vi "test - Add VI Reference Script.vi"(8 "error in (no error)":errorcluster, 11 "TestCase in":refnum<class "testcase-csmhelper.lvclass">) -> (0 "error out":errorcluster, 3 "TestCase out":refnum<class "testcase-csmhelper.lvclass">)   [LabVIEW 2017, in "testcase-csmhelper.lvclass"]
uses:
  testcase-csmhelper.lvclass
  src/user.lib/_NEVSTOP/Communicable State Machine(CSM)/_csmHelper/CSM-Helper.lvclass/CSM-Helper.ctl
  src/user.lib/_NEVSTOP/Communicable State Machine(CSM)/_csmHelper/Properties/Read VI Ref.vi
  src/user.lib/_NEVSTOP/Communicable State Machine(CSM)/_csmHelper/API/Create From VI Reference.vi
  src/user.lib/_NEVSTOP/Communicable State Machine(CSM)/_csmHelper/API/Open Block Diagram.vi
  src/user.lib/_NEVSTOP/Communicable State Machine(CSM)/_csmHelper/API/Start Undo.vi
  src/user.lib/_NEVSTOP/Communicable State Machine(CSM)/_csmHelper/API/Remove State Frame.vi
  src/user.lib/_NEVSTOP/Communicable State Machine(CSM)/_csmHelper/usecase/Add VI Reference Case.vi
  src/user.lib/_NEVSTOP/Communicable State Machine(CSM)/_csmHelper/API/Stop Undo.vi
  src/user.lib/_NEVSTOP/Communicable State Machine(CSM)/_csmHelper/Properties/Read States.vi
  src/user.lib/_NEVSTOP/Communicable State Machine(CSM)/_csmHelper/API/Undo.vi
  src/user.lib/_NEVSTOP/Communicable State Machine(CSM)/_csmHelper/API/Destroy.vi
  <vilib>/addons/_JKI Toolkits/VI Tester/TestCase.llb/TestCase.lvclass
  src/user.lib/_NEVSTOP/Communicable State Machine(CSM)/_csmHelper/CSM-Helper.lvclass
  C:/Program Files (x86)/National Instruments/LabVIEW 2017/vi.lib/addons/_JKI Toolkits/VI Tester/TestCase.llb/TestCase.lvclass
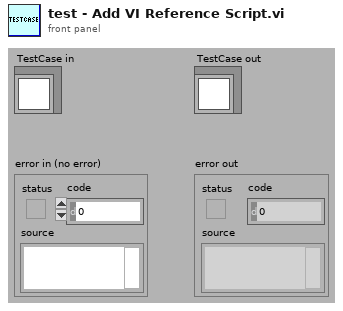
[diagram p1: front panel]
types:
  T1 = enum32{"Bad", "Idle", "Run top level", "Running"}
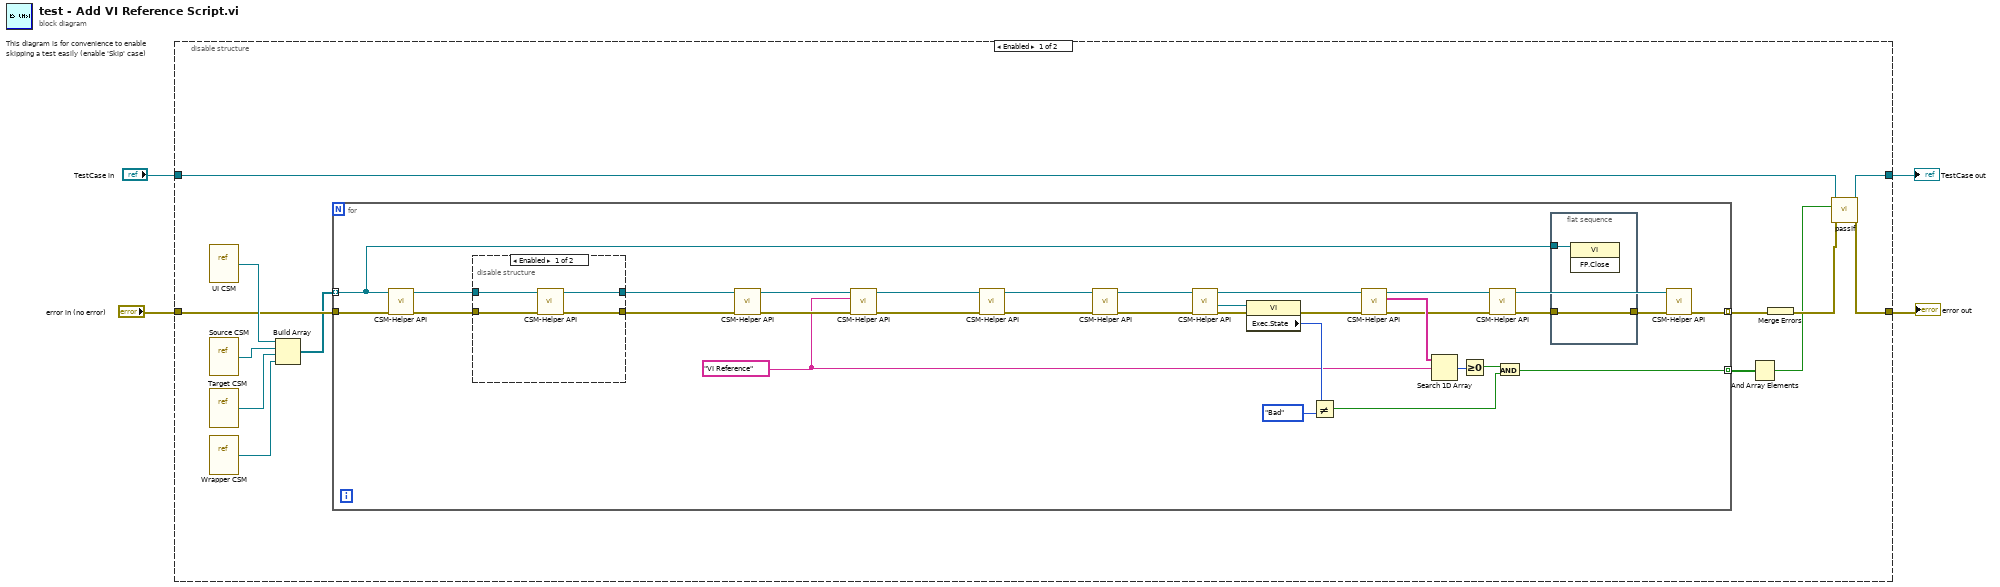
[diagram p0: block diagram]
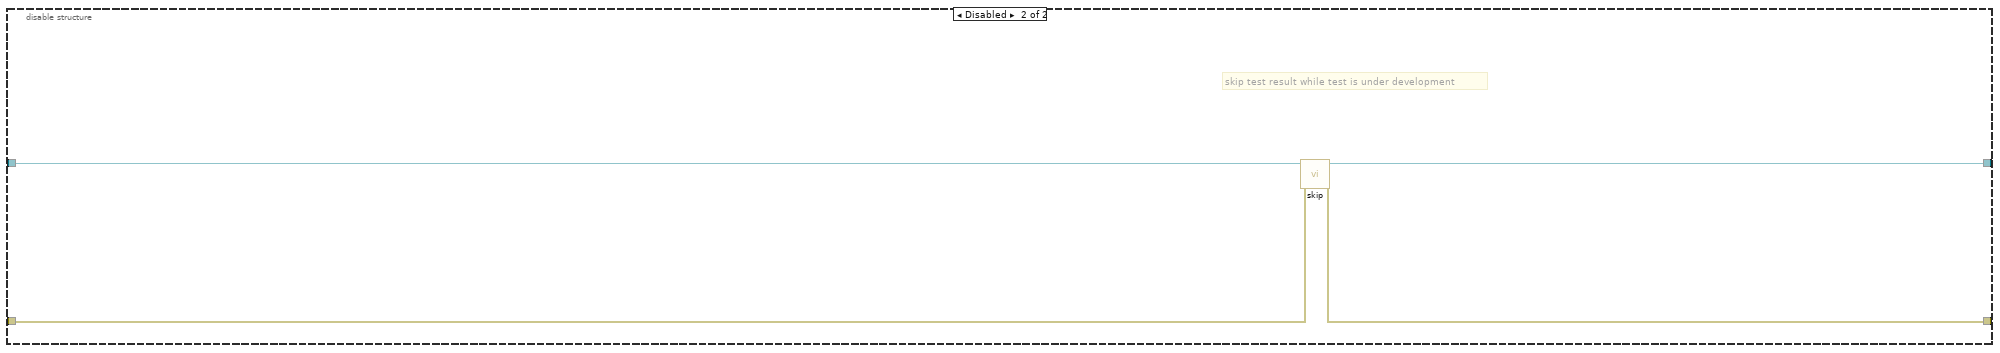
[diagram p3: hidden frame]
diagram:
  n1 = disable-structure "This diagram is for convenience to enable skipping a test easily (enable 'Skip' case)" shown="Enabled" {
    disable-tunnel: "TestCase in" -> [w17 w61]
    disable-tunnel: [w16 w59] -> w1
    disable-tunnel: [w15 w60] -> w3
    disable-tunnel: "error in (no error)" -> [w12 w58]
    frame Enabled {
      n2 = vi-ref "UI CSM.vi"() -> (w14:refnum<vi>)
      n3 = vi-ref "Source CSM.vi"() -> (w8:refnum<vi>)
      n4 = vi-ref "Target CSM.vi"() -> (w7:refnum<vi>)
      n5 = vi-ref "Wrapper CSM.vi"() -> (w6:refnum<vi>)
      n6 = Build Array(w14, w8, w7, w6) -> (w5:refnum<vi>[])
      n7 = for {
        tunnel: w5 -> [w20] mode=indexing
        tunnel: [w49] -> w13 mode=indexing
        tunnel: w12 -> [w48]
        tunnel: [w47] -> w11 mode=indexing
        w21 = "VI Reference" ("element")
        n8 = call-poly "CSM-Helper API.vi"("error in (no error)"=w48, "VI"=w20) -> ("error out"=w25:errorcluster, "CSM-Helper.lvclass"=w24:refnum<class "CSM-Helper.lvclass">)  [unwired: 8 in]
        n9 = disable-structure shown="Enabled" {
          disable-tunnel: w25 -> [w55 w56]
          disable-tunnel: w24 -> [w54 w57]
          disable-tunnel: [w53 w56] -> w23
          disable-tunnel: [w52 w57] -> w22
          frame Enabled {
            n10 = call-poly "CSM-Helper API.vi"("error in (no error)"=w55, "CSM-Helper in"=w54) -> ("error out"=w53:errorcluster, "CSM-Helper out"=w52:refnum<class "CSM-Helper.lvclass">)  [unwired: 8 in]
          }
          frame Disabled {
          }
        }
        n11 = call-poly "CSM-Helper API.vi"("error in (no error)"=w23, "CSM-Helper in"=w22) -> ("error out"=w26:errorcluster, "CSM-Helper out"=w27:refnum<class "CSM-Helper.lvclass">)  [unwired: 8 in]
        n12 = call-poly "CSM-Helper API.vi"("error in (no error)"=w26, "element"=w21, "CSM-Helper in"=w27) -> ("error out"=w29:errorcluster, "CSM-Helper out"=w28:refnum<class "CSM-Helper.lvclass">)  [unwired: 7 in]
        n13 = call-poly "CSM-Helper API.vi"("error in"=w29, "CSM-Helper in"=w28) -> ("error out"=w44:errorcluster, "CSM-Helper out"=w45:refnum<class "CSM-Helper.lvclass">)  [unwired: 8 in]
        n14 = call-poly "CSM-Helper API.vi"("error in (no error)"=w44, "CSM-Helper in"=w45) -> ("error out"=w43:errorcluster, "CSM-Helper out"=w42:refnum<class "CSM-Helper.lvclass">)  [unwired: 8 in]
        n15 = call-poly "CSM-Helper API.vi"("error in (no error)"=w43, "CSM-Helper in"=w42) -> ("error out"=w41:errorcluster, "VI"=w40:refnum<vi>, "CSM-Helper out"=w33:refnum<class "CSM-Helper.lvclass">)  [unwired: 7 in]
        n16 = property class="VI"(reference=w40, error in=w41) -> (error out=w34:errorcluster, "Exec.State"=w39:T1)  [unwired: 1 out]
        n17 = Not Equal?(x=w39, y=T1."Bad") -> (x != y?=w37:bool)
        n18 = call-poly "CSM-Helper API.vi"("error in (no error)"=w34, "CSM-Helper in"=w33) -> ("error out"=w30:errorcluster, "Value"=w35:string[], "CSM-Helper out"=w31:refnum<class "CSM-Helper.lvclass">)  [unwired: 7 in]
        n19 = Search 1D Array(1D array=w35, element=w21) -> (index of element=w36:i32)  [unwired: 1 in]
        n20 = Greater Or Equal To 0?(x=w36) -> (x >= 0?=w32:bool)
        n21 = call-poly "CSM-Helper API.vi"("error in (no error)"=w30, "CSM-Helper in"=w31) -> ("error out"=w18:errorcluster, "CSM-Helper out"=w46:refnum<class "CSM-Helper.lvclass">)  [unwired: 8 in]
        n22 = And(x=w32, y=w37) -> (x .and. y?=w49:bool)
        n23 = flat-sequence {
          tunnel: w20 -> [w51]
          tunnel: [w50] -> w19
          tunnel: w18 -> [w50]
          frame #0 {
            n24 = invoke class="VI" method="FP.Close"(reference=w51) -> ()  [unwired: 2 in, 3 out]
          }
        }
        n25 = call-poly "CSM-Helper API.vi"("error in (no error)"=w19, "CSM-Helper in"=w46) -> ("error out"=w47:errorcluster)  [unwired: 8 in, 1 out]
      }
      n26 = And Array Elements(Boolean array=w13) -> (logical AND=w9:bool)
      n27 = Merge Errors(w11) -> (w10:errorcluster)
      n28 = call-dynamic "passIf.vi"("error in (no error)"=w10, "pass"=w9, "TestCase in"=w17) -> ("error out"=w15:errorcluster, "TestCase out"=w16:refnum<class "testcase-csmhelper.lvclass">)  [unwired: 7 in]
    }
    frame Disabled {
      # "skip test result while test is under development"
      n29 = call <vilib>:"skip.vi"("error in (no error)"=w58, "TestCase in"=w61) -> ("error out"=w60:errorcluster, "TestCase out"=w59:refnum<class "testcase-csmhelper.lvclass">)  [unwired: 8 in]
    }
  }
  "error out" <- w3
  "TestCase out" <- w1
